vi "FPGA_AIReadOffset.vi"(8 "error in (no error)":errorcluster, 10 "Channel":T1, 11 "AI Reference":T2) -> (0 "error out":errorcluster, 2 "Offset":i32, 3 "AI Reference":T2)   [LabVIEW 2017]
uses:
  <vilib>/Rock Robotics/SystemInterfaces/AI/FPGA_AIDevRef.ctl
  <vilib>/Rock Robotics/SystemInterfaces/AI/FPGA_AIChannel.ctl
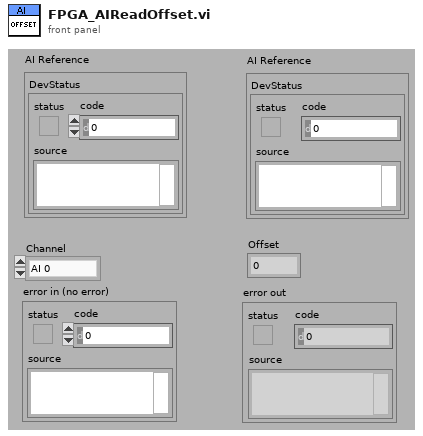
[diagram p1: front panel]
types:
  T1 = typedef "FPGA_AIChannel.ctl" = enum8{"AI 0", "AI 1", "AI 2", "AI 3", "AI MXP 0", "AI MXP 1", "AI MXP 2", "AI MXP 3", "Invalid"}
  T2 = typedef "FPGA_AIDevRef.ctl" = cluster{"DevStatus":errorcluster}
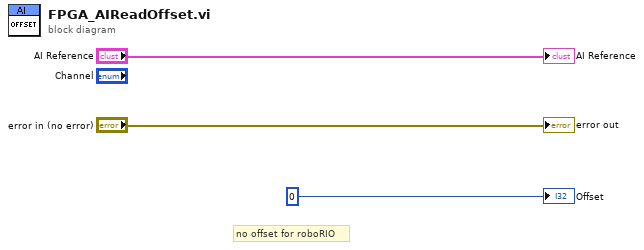
[diagram p0: block diagram]
diagram:
  # "no offset for roboRIO"
  "AI Reference" <- "AI Reference"
  "Offset" <- 0 ("Offset")
  "error out" <- "error in (no error)"
